vi "FRC3005_GyroXRS450_Open.vi"(8 "error in (no error)":errorcluster, 10 "Sample Rate (ms)":dbl=1.0, 11 "SPI Bus":T3) -> (0 "error out":errorcluster, 3 "GyroDeviceRef":T1 {"Sample Rate" min=0.25 max=100.0 step=0.25})   [LabVIEW 2016, in "Path Track.lvlib"]
uses:
  Path Track.lvlib
  <vilib>/Rock Robotics/SystemInterfaces/spilib/spi_bus.ctl
  <vilib>/Rock Robotics/WPI/Gyro/WPI_GyroDevRef.ctl
  <vilib>/Rock Robotics/SystemInterfaces/AI/FPGA_AIChannel.ctl
  <vilib>/Rock Robotics/WPI/SPI/WPI_SPIMode.ctl
  <vilib>/Rock Robotics/WPI/Gyro/ADXRS453/WPI_Gyro_ADXRS453_Registers.ctl
  <vilib>/Rock Robotics/SystemInterfaces/NetworkCommunication/NetComm_UsageReport_ResourceType.ctl
panel:
  # "Analog"
  # "XRS"
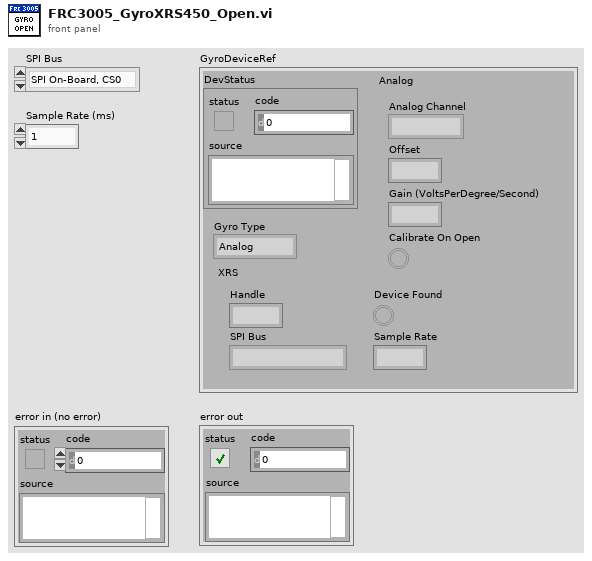
[diagram p1: front panel]
types:
  T1 = typedef "WPI_GyroDevRef.ctl" = cluster{"DevStatus":errorcluster, "Analog Channel":T2, "Offset":dbl, "Gain (VoltsPerDegree/Second)":dbl, "Gyro Type":enum16{"Analog", "XRS450"}, "Handle":i32, "SPI Bus":T3, "Device Found":bool, "Sample Rate":dbl, "Calibrate On Open":bool}
  T2 = typedef "FPGA_AIChannel.ctl" = enum8{"AI 0", "AI 1", "AI 2", "AI 3", "AI MXP 0", "AI MXP 1", "AI MXP 2", "AI MXP 3", "Invalid"}
  T3 = typedef "spi_bus.ctl" = enum16{"SPI On-Board, CS0", "SPI On-Board, CS1", "SPI On-Board, CS2", "SPI On-Board, CS3", "SPI MXP", "Invalid"}
  T4 = typedef "WPI_SPIMode.ctl" = enum16{"Mode 0 (Clk Idle Low,Sample on Leading)", "Mode 1 (Clk Idle Low,Sample on Trailing)", "Mode 2 (Clk Idle High,Sample on Leading)", "Mode 3 (Clk Idle High,Sample on Trailing)"}
  T5 = typedef "NetComm_UsageReport_ResourceType.ctl" = enum8{"Controller", "Module", "Language", "CANPlugin", "Accelerometer", "ADXL345", "AnalogChannel", "AnalogTrigger", "AnalogTriggerOutput", "CANJaguar", "Compressor", "Counter", "Dashboard", "DigitalInput", "DigitalOutput", "DriverStationCIO", "DriverStationEIO", "DriverStationLCD", "Encoder", "GearTooth", "Gyro", "I2C", "Framework", "Jaguar", "Joystick", "Kinect", "KinectStick", "PIDController", "Preferences", "PWM", "Relay", "RobotDrive", "SerialPort", "Servo", "Solenoid", "SPI", "Task", "Ultrasonic", "Victor", "Button", "Command", "AxisCamera", "PCVideoServer", "SmartDashboard", "Talon", "HiTechnicColorSensor", "HiTechnicAccel", "HiTechnicCompass", "SRF08", "AnalogOutput", "Victor SP", "Talon SRX", "CAN Talon SRX", "ADXL362 Accel", "ADXRS450 Gyro", "Rev SPARK", "Mindsensors SD540", "Digital Filter", "ADIS16448", "PDP", "PCM", "PigeonIMU"}
  T6 = typedef "WPI_Gyro_ADXRS453_Registers.ctl" = u16
  T7 = typedef "WPI_SPIDevRef.ctl" = cluster{"DevStatus":errorcluster, "Handle":i32, "SPI Bus":T3}
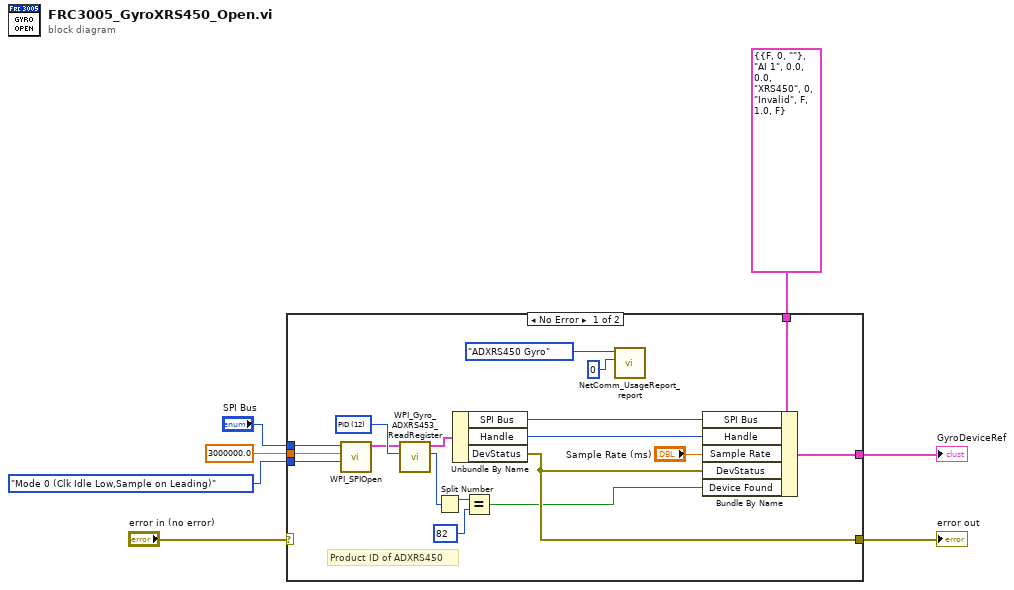
[diagram p0: block diagram]
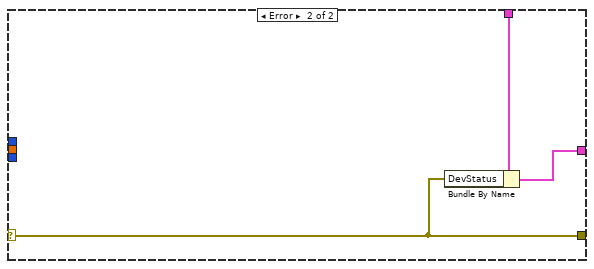
[diagram p2: hidden frame]
diagram:
  n1 = case shown="No Error" "error in (no error)" {
    selector: "error in (no error)" -> [_ w27]
    tunnel: "SPI Bus" -> [w25 _]
    tunnel: 3000000.0 ("Clock Rate (Hz)") -> [w24 _]
    tunnel: WPI_SPIMode."Mode 0 (Clk Idle Low,Sample on Leading)" ("Mode (3)") -> [w23 _]
    tunnel: [w18 w27] -> w5
    tunnel: T1 {"DevStatus"={"status"=FALSE, "code"=0, "source"=""}, "Analog Channel"=enum."AI 1", "Offset"=0.0, "Gain (VoltsPerDegree/Second)"=0.0, "Gyro Type"=enum."XRS450", "Handle"=0, "SPI Bus"=enum."Invalid", "Device Found"=FALSE, "Sample Rate"=1.0, "Calibrate On Open"=FALSE} ("GyroDeviceRef") -> [w22 w28]
    tunnel: [w19 w26] -> w7
    frame No Error {
      w16 = T6 12 items=["Rate"=0, "Tem"=2, "LoCST"=4, "HiCST"=6, "Quad"=8, "Fault"=10, "PID"=12, "SN High"=14, "SN Low"=16]
      # "Product ID of ADXRS450"
      n2 = call <vilib>:"WPI_SPIOpen.vi"("Mode (3)"=w23, "Clock Rate (Hz)"=w24, "SPI Bus"=w25) -> ("SPIDevRef"=w12:T7)  [unwired: 7 in, 1 out]
      n3 = call <vilib>:"WPI_Gyro_ADXRS453_ReadRegister.vi"("ADXRS453 Register"=w16, "SPIDevRef in"=w12) -> ("Register Value"=w15:u16, "SPIDevRef out"=w11:T7)  [unwired: 7 in, 1 out]
      n4 = Split Number(x=w15) -> (hi(x)=w14:u8)  [unwired: 1 out]
      n5 = Unbundle By Name(w11) -> ("SPI Bus"=w21:T3, "Handle"=w20:i32, "DevStatus"=w18:errorcluster)
      n6 = Equal?(x=w14, y=u8 82) -> (x = y?=w10:bool)
      n7 = call <vilib>:"NetComm_UsageReport_report.vi"("Instance Number"=u8 0, "Resource Type"=NetComm_UsageReport_ResourceType."ADXRS450 Gyro") -> ()  [unwired: 10 in]
      n8 = Bundle By Name(cluster=w22, "SPI Bus"=w21, "Handle"=w20, "Sample Rate"="Sample Rate (ms)", "DevStatus"=w18, "Device Found"=w10) -> (w19:T1)
    }
    frame Error {
      n9 = Bundle By Name(cluster=w28, "DevStatus"=w27) -> (w26:T1)
    }
  }
  "GyroDeviceRef" <- w7
  "error out" <- w5
